vi "saturatore_unipolare_progressivo.vi"(1 "waveform":waveform(dbl), 2 "V*":dbl min=0.0, 3 "Vfs":dbl min=0.0) -> (0 "output waveform":waveform(dbl))   [LabVIEW 2009]
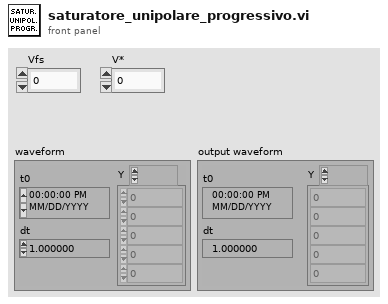
[diagram p1: front panel]
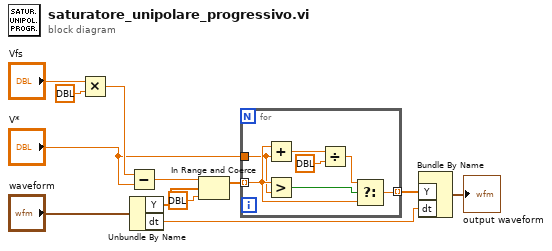
[diagram p0: block diagram]
diagram:
  n1 = Multiply(x="Vfs", y=dbl ?) -> (x*y=w5:dbl)
  n2 = Subtract(x=w5, y="V*") -> (x-y=w4:dbl)
  n3 = Unbundle By Name("waveform") -> ("Y"=w8:dbl[], "dt"=w11:dbl)
  n4 = In Range and Coerce(upper limit=w4, x=w8, lower limit=dbl ?) -> (coerced(x)=w3:dbl[])  [unwired: 1 out]
  n5 = for {
    tunnel: w3 -> [w18] mode=indexing
    tunnel: "V*" -> [w17]
    tunnel: [w13] -> w1 mode=indexing
    n6 = Add(x=w18, y=w17) -> (x+y=w16:dbl)
    n7 = Greater?(x=w18, y=w17) -> (0:w19:bool)
    n8 = Divide(x=w16, y=dbl ?) -> (x/y=w14:dbl)
    n9 = Select(t=w14, s=w19, f=w18) -> (s? t:f=w13:dbl)
  }
  n10 = Bundle By Name("Y"=w1, "dt"=w11) -> (→"output waveform":waveform(dbl))  [unwired: 1 in]
